vi "getState.vi"(8 "error in (no error)":errorcluster, 11 "ReadyState in":refnum<class "ReadyState.lvclass">) -> (0 "error out":errorcluster, 2 "State":T1, 3 "ReadyState out":refnum<class "ReadyState.lvclass">)   [LabVIEW 2016, in "ReadyState.lvclass"]
uses:
  ReadyState.lvclass
  internalState.ctl
  Electrometer.lvclass
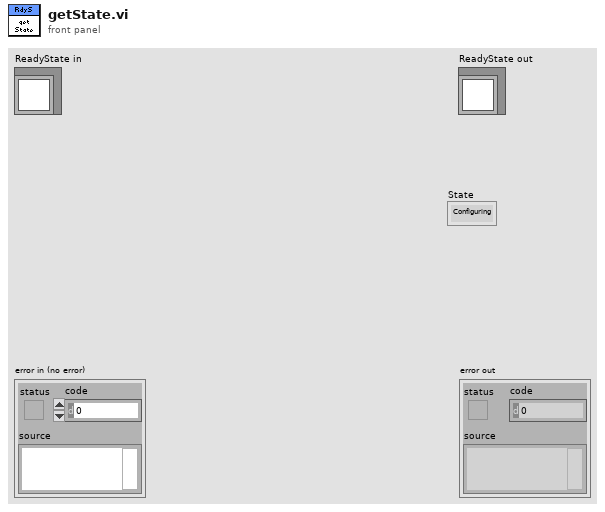
[diagram p1: front panel]
types:
  T1 = typedef "Electrometer.lvclass/internalState.ctl" = enum16{"Configuring", "Ready", "Reading"}
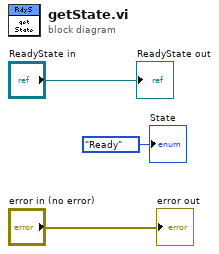
[diagram p0: block diagram]
diagram:
  "error out" <- "error in (no error)"
  "ReadyState out" <- "ReadyState in"
  "State" <- internalState."Ready" ("State")
